vi "(SubVI) Sine Generator_YCC.vi"(4 "Points to be generated":i32, 5 "fs (Hz)":dbl, 7 "initial position (um)":dbl, 8 "Amplitude, A (nm)":dbl, 9 "f_drive (Hz)":dbl) -> (0 "Total Need time (s)":dbl format="%.5f", 1 "waiting time (to write) (ms)":dbl, 2 "Position Array (um)":dbl[](array[numeric]), 3 "Time Array (s)":dbl[](array[numeric]))   [LabVIEW 2014]
panel:
  out "XY Graph":cluster{dbl[], dbl[]}(graph)
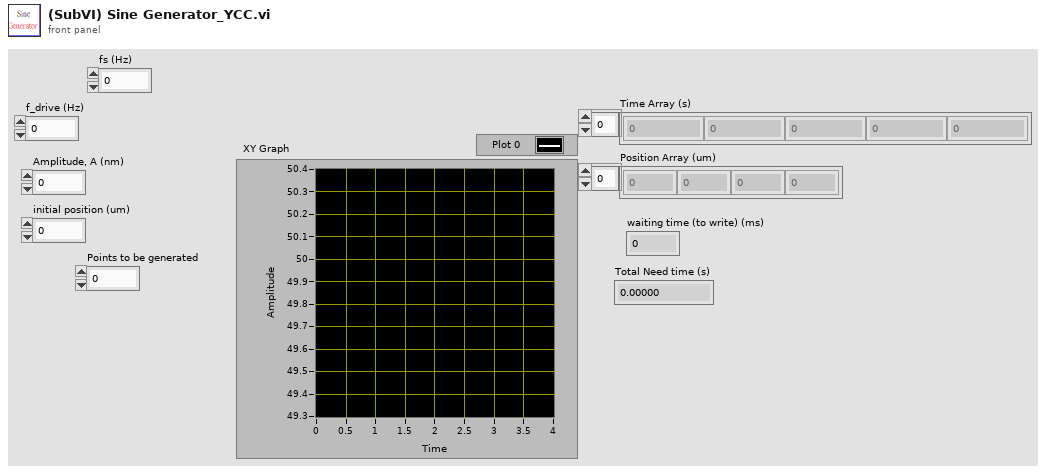
[diagram p1: front panel]
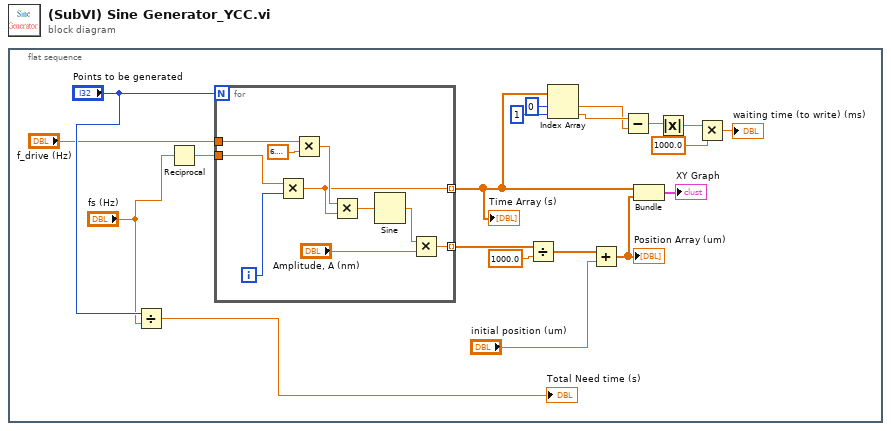
[diagram p0: block diagram]
diagram:
  n1 = flat-sequence {
    frame #0 {
      n2 = Divide(x="Points to be generated", y="fs (Hz)") -> (x/y=→"Total Need time (s)":dbl)
      n3 = Reciprocal(x="fs (Hz)") -> (1/x=w20:dbl)
      n4 = for {
        N: "Points to be generated" -> [_]
        tunnel: "f_drive (Hz)" -> [w29]
        tunnel: w20 -> [w28]
        tunnel: [w22] -> w18 mode=indexing
        tunnel: [w25] -> w9 mode=indexing
        i -> [w21]
        n5 = Multiply(x=w28, y=w21) -> (x*y=w25:dbl)
        n6 = Multiply(x=w29, y=6.283185307179586) -> (x*y=w27:dbl)
        n7 = Multiply(x=w27, y=w25) -> (x*y=w26:dbl)
        n8 = Sine(x=w26) -> (sin(x)=w24:dbl)
        n9 = Multiply(x=w24, y="Amplitude, A (nm)") -> (x*y=w22:dbl)
      }
      "Time Array (s)" <- w9
      n10 = Divide(x=w18, y=1000.0) -> (x/y=w16:dbl[])
      n11 = Index Array(array=w9, index #1=0 ("index"), index #2=1 ("index")) -> (element #1=w5:dbl, element #2=w6:dbl)
      n12 = Add(x=w16, y="initial position (um)") -> (x+y=w14:dbl[])
      "Position Array (um)" <- w14
      n13 = Subtract(x=w6, y=w5) -> (x-y=w4:dbl)
      n14 = Bundle(w9, w14) -> (→"XY Graph":cluster{dbl[], dbl[]})  [unwired: 1 in]
      n15 = Absolute Value(x=w4) -> (abs(x)=w3:dbl)
      n16 = Multiply(x=w3, y=1000.0) -> (x*y=→"waiting time (to write) (ms)":dbl)
    }
  }
